vi "_stop_measure.vi"(8 "error in (no error)":errorcluster, 11 "UV-VIS_AVANTES in":refnum<class "UV-VIS_AVANTES.lvclass">) -> (0 "error out":errorcluster, 3 "UV-VIS_AVANTES out":refnum<class "UV-VIS_AVANTES.lvclass">)   [LabVIEW 2020, in "UV-VIS_AVANTES.lvclass"]
uses:
  UV-VIS_AVANTES.lvclass
  C:/dev/TRANCON/Classes/Detector/Detector.lvclass
  Detector.lvclass/Detector.ctl
  UV-VIS_AVANTES.lvclass/UV-VIS_AVANTES.ctl
  Detector.lvclass
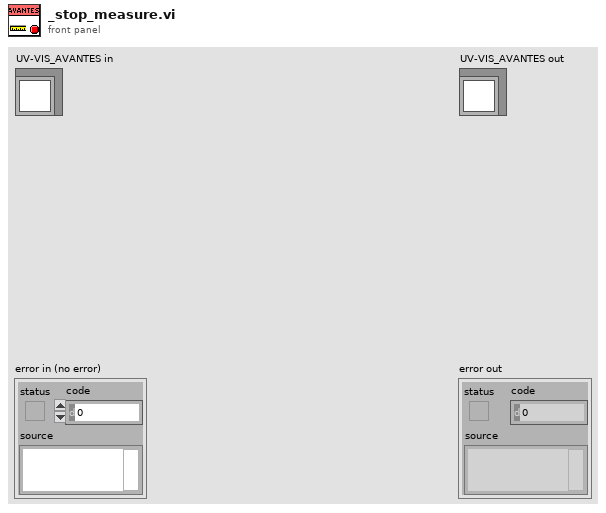
[diagram p1: front panel]
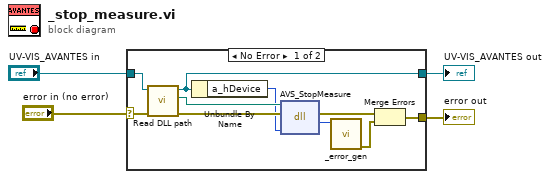
[diagram p0: block diagram]
diagram:
  n1 = case shown="No Error" "error in (no error)" {
    selector: "error in (no error)" -> [w13 w16]
    tunnel: [w7 w16] -> w3
    tunnel: [w10 w15] -> w1
    tunnel: "UV-VIS_AVANTES in" -> [w14 w15]
    frame No Error {
      n2 = call "Read DLL path.vi"("error in (no error)"=w13, "Detector in"=w14) -> ("error out"=w12:errorcluster, "DLL path"=w11:path, "Detector out"=w10:refnum<class "UV-VIS_AVANTES.lvclass">)  [unwired: 7 in]
      n3 = Unbundle By Name(w10) -> ("a_hDevice"=w9:i32)
      n4 = dll-call lib="C:/AvaSpecX64-DLL_9.4/examples/LabView/LabViewSingleChan/avaspec.dll" fn="AVS_StopMeasure"(path in=w11, error in=w12, "a_hDevice"=w9) -> (error out=w6:errorcluster, "return type"=w5:i32)  [unwired: 2 in, 1 out]
      n5 = call "_error_gen.vi"("return type"=w5) -> ("error out"=w8:errorcluster)  [unwired: 10 in]
      n6 = Merge Errors(w6, w8) -> (w7:errorcluster)
    }
    frame Error {
    }
  }
  "error out" <- w3
  "UV-VIS_AVANTES out" <- w1
